vi "ActionVIOnSave.vi"(8 "error in (no error)":errorcluster, 11 "Device Item Ref in":T1 format="%.0x") -> (0 "error out":errorcluster, 3 "Device Item Ref out":T1 format="%.0x")   [LabVIEW 2017, in "DSF System Explorer.lvlib"]
uses:
  DSF System Explorer.lvlib
  <vilib>/NI Veristand/Custom Device API/Custom Device Item Ref.ctl
  <vilib>/NI Veristand/Custom Device API/Custom Device API.lvlib
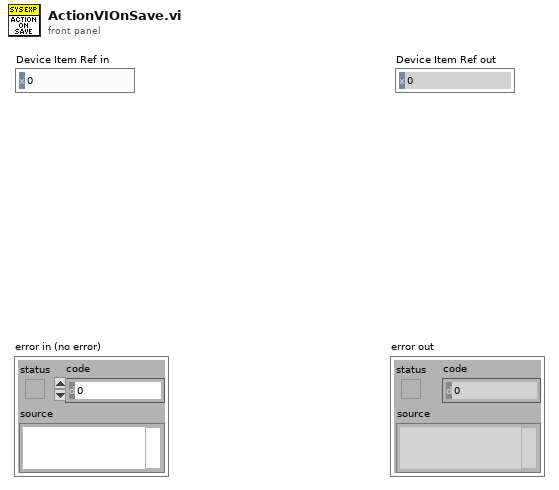
[diagram p1: front panel]
types:
  T1 = typedef "Custom Device API.lvlib/Custom Device Item Ref.ctl" = u64
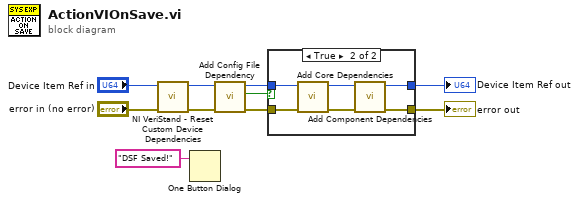
[diagram p0: block diagram]
diagram:
  n1 = call <vilib>:"NI VeriStand - Reset Custom Device Dependencies.vi"("error in (no error)"="error in (no error)", "Device Ref in"="Device Item Ref in") -> ("error out"=w3:errorcluster, "Device Ref out"=w4:T1)  [unwired: 8 in]
  n2 = One Button Dialog(message="DSF Saved!") -> ()  [unwired: 1 in, 1 out]
  n3 = call "Add Config File Dependency.vi"("error in (no error)"=w3, "Item Ref in"=w4) -> ("error out"=w7:errorcluster, "configuration file set?"=w2:bool, "Device Ref out"=w8:T1)  [unwired: 7 in]
  n4 = case shown="True" w2 {
    tunnel: [w12 w18] -> w10
    tunnel: [w11 w17] -> w9
    tunnel: w8 -> [w12 w14]
    tunnel: w7 -> [w11 w13]
    frame False {
    }
    frame True {
      n5 = call "Add Core Dependencies.vi"("error in (no error)"=w13, "Item Ref in"=w14) -> ("error out"=w15:errorcluster, "Device Ref out"=w16:T1)  [unwired: 8 in]
      n6 = call "Add Component Dependencies.vi"("error in (no error)"=w15, "Device Item Ref in"=w16) -> ("error out"=w17:errorcluster, "Device Ref out"=w18:T1)  [unwired: 7 in, 1 out]
    }
  }
  "error out" <- w9
  "Device Item Ref out" <- w10
